vi "(4) Encoder Version Position.vi"() -> ()   [LabVIEW 2020]
uses:
  <instrlib>/Arcus Ethernet Driver 1.0.0/ArcusEthernetComm/classes/Controller/_Controller.lvclass
panel:
  out "Z Response":string
  out "Y Response":string
  out "X Response":string
  in  "Get Response":bool
  out "Scanning Rig Disconnection":errorcluster={"status"=TRUE, "code"=0, "source"=""}
  in  "error in (no error)":errorcluster
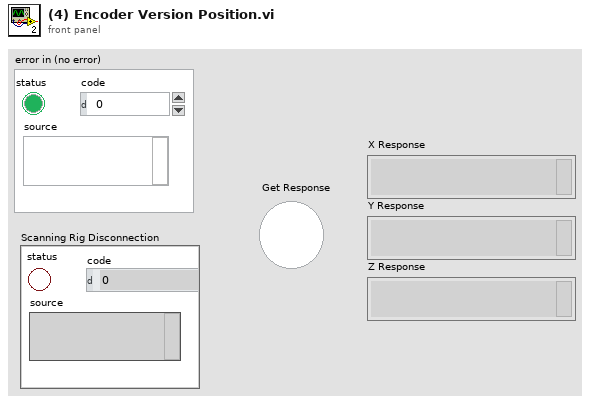
[diagram p1: front panel]
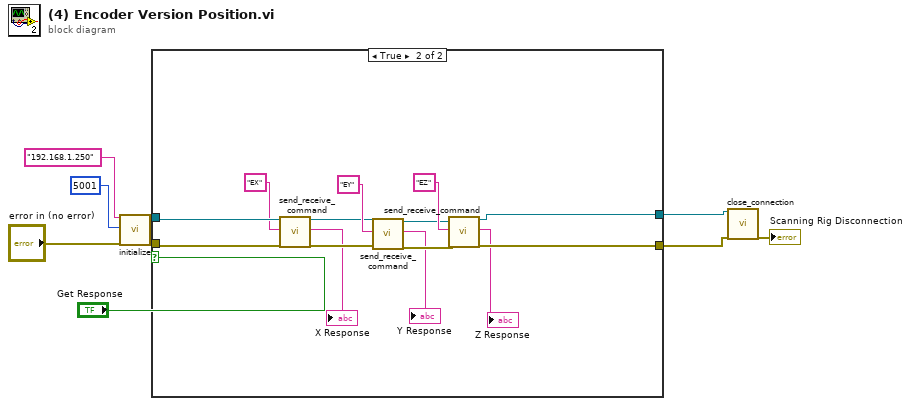
[diagram p0: block diagram]
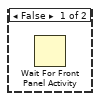
[diagram p2: hidden frame]
diagram:
  n1 = call <instrlib>:"initialize.vi"("ip_address (in)"="192.168.1.250", "dev_port(def=5001)"=u16 5001, "error in (no error)"="error in (no error)") -> ("reference (out)"=w5:refnum<class "_Controller.lvclass">, "error out"=w4:errorcluster)  [unwired: 15 in]
  n2 = case shown="True" "Get Response" {
    tunnel: w5 -> [_ w23]
    tunnel: w4 -> [_ w22]
    tunnel: [_ w14] -> w2
    tunnel: [_ w13] -> w1
    frame False {
      n3 = Wait For Front Panel Activity() -> ()  [unwired: 3 in, 1 out]
    }
    frame True {
      n4 = call <instrlib>:"send_receive_command.vi"("reference (in)"=w23, "ASCII Command (in)"="EX", "error in (no error)"=w22) -> ("reference (out)"=w19:refnum<class "_Controller.lvclass">, "response (out)"=→"X Response":string, "error out"=w18:errorcluster)  [unwired: 12 in, 2 out]
      n5 = call <instrlib>:"send_receive_command.vi"("reference (in)"=w19, "ASCII Command (in)"="EY", "error in (no error)"=w18) -> ("reference (out)"=w16:refnum<class "_Controller.lvclass">, "response (out)"=→"Y Response":string, "error out"=w15:errorcluster)  [unwired: 12 in, 2 out]
      n6 = call <instrlib>:"send_receive_command.vi"("reference (in)"=w16, "ASCII Command (in)"="EZ", "error in (no error)"=w15) -> ("reference (out)"=w14:refnum<class "_Controller.lvclass">, "response (out)"=→"Z Response":string, "error out"=w13:errorcluster)  [unwired: 12 in, 2 out]
    }
  }
  n7 = call <instrlib>:"close_connection.vi"("reference (in)"=w2, "error in (no error)"=w1) -> ("error out"=→"Scanning Rig Disconnection":errorcluster)  [unwired: 16 in, 1 out]
